vi "Delete_Data.vi"(8 "error in (no error)":errorcluster, 10 "day":i32, 11 "DBlink":string="Driver={ODBC Driver 17 for SQL Server};Server=localhost\\SQLEXPRESS;Database=AADXB08;UID=labview;PWD=Dsa@54137926") -> (0 "error out":errorcluster)   [LabVIEW 2019]
uses:
  <vilib>/addons/database/Connection.llb/DB Tools Open Connec (String).vi
  <vilib>/addons/database/NI_Database_API.lvlib
panel:
  out "concatenated string":string="where create_time between '2022-2-14' AND '2022-2-14 23:59:59'"
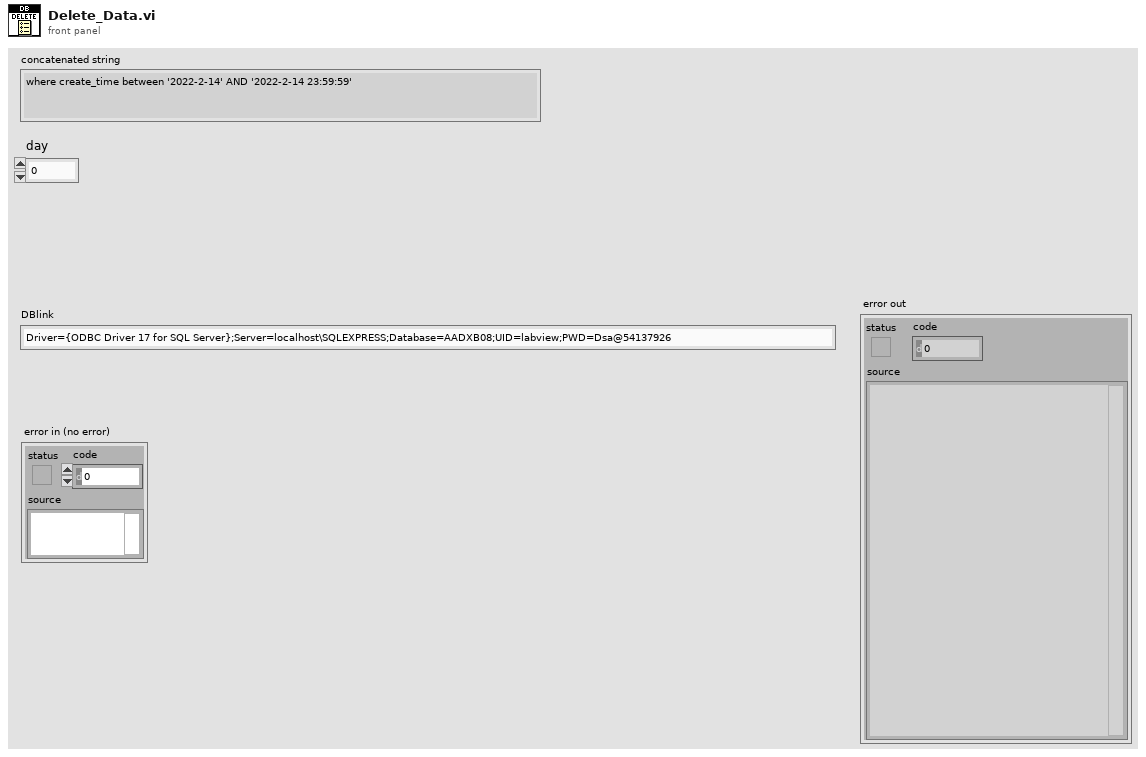
[diagram p1: front panel]
types:
  T1 = typedef "NI_Database_API.lvlib/Conn ObjectReference.ctl" = refnum<k1>
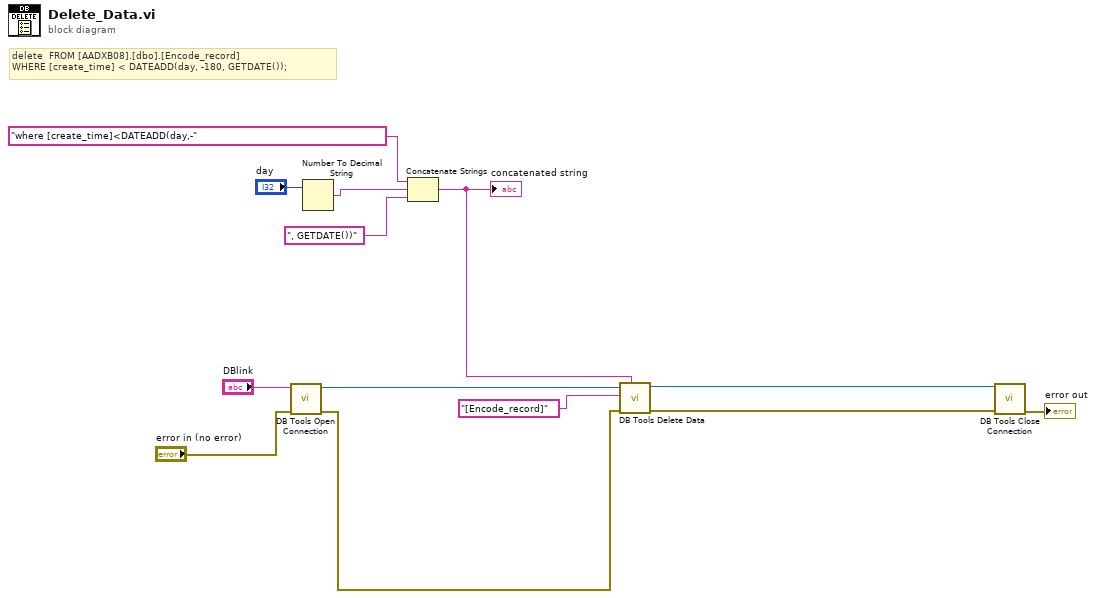
[diagram p0: block diagram]
diagram:
  # "delete  FROM [AADXB08].[dbo].[Encode_record]\nWHERE [create_time] < DATEADD(day, -180, GETDATE());"
  n1 = call-poly <vilib>:"DB Tools Open Connection.vi"("error in (no error)"="error in (no error)", "connection information"="DBlink") -> ("error out"=w7:errorcluster, "connection reference"=w9:T1)  [unwired: 6 in]
  n2 = Number To Decimal String(number="day") -> (decimal integer string=w4:string)  [unwired: 1 in]
  n3 = Concatenate Strings("where [create_time]<DATEADD(day,-" ("format string"), w4, ", GETDATE())" ("string")) -> (w1:string)
  "concatenated string" <- w1
  n4 = call <vilib>:"DB Tools Delete Data.vi"("condition"=w1, "error in (no error)"=w7, "table"="[Encode_record]", "connection reference"=w9) -> ("error out"=w6:errorcluster, "connection reference out"=w5:T1)  [unwired: 6 in]
  n5 = call <vilib>:"DB Tools Close Connection.vi"("error in (no error)"=w6, "connection reference"=w5) -> ("error out"=→"error out":errorcluster)  [unwired: 5 in]
